vi "TCP.IP Server for Ripple Detection_requirements.vi"() -> ()   [LabVIEW 2021]
doc: "Demonstrates how to set up a basic TCP connection, send data to the specified port once a connection has been established, and terminate the connection once the data has been sent. This VI is designed to stop if the TCP connection is terminated. The data sent in this example is an array of random numbers."
panel:
  out "size":i64 format="%.6p"
  out "error IO":errorcluster
  in  "Number of row to read \nat a time":i32=10000
  in  "File Path":path
  out "Iteration terminal":i32
  in  "Stop 2":bool
  in  "Client Closed":string="The client VI closed the connection."
  in  "Stop":bool
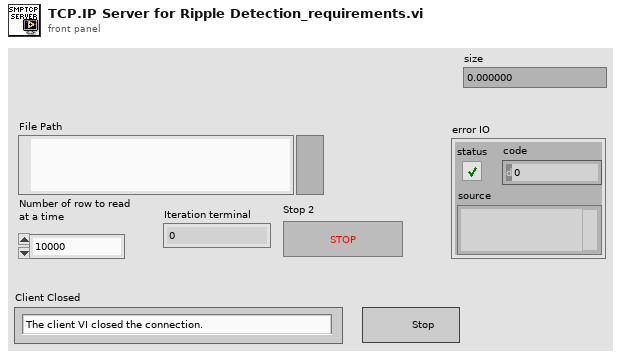
[diagram p1: front panel]
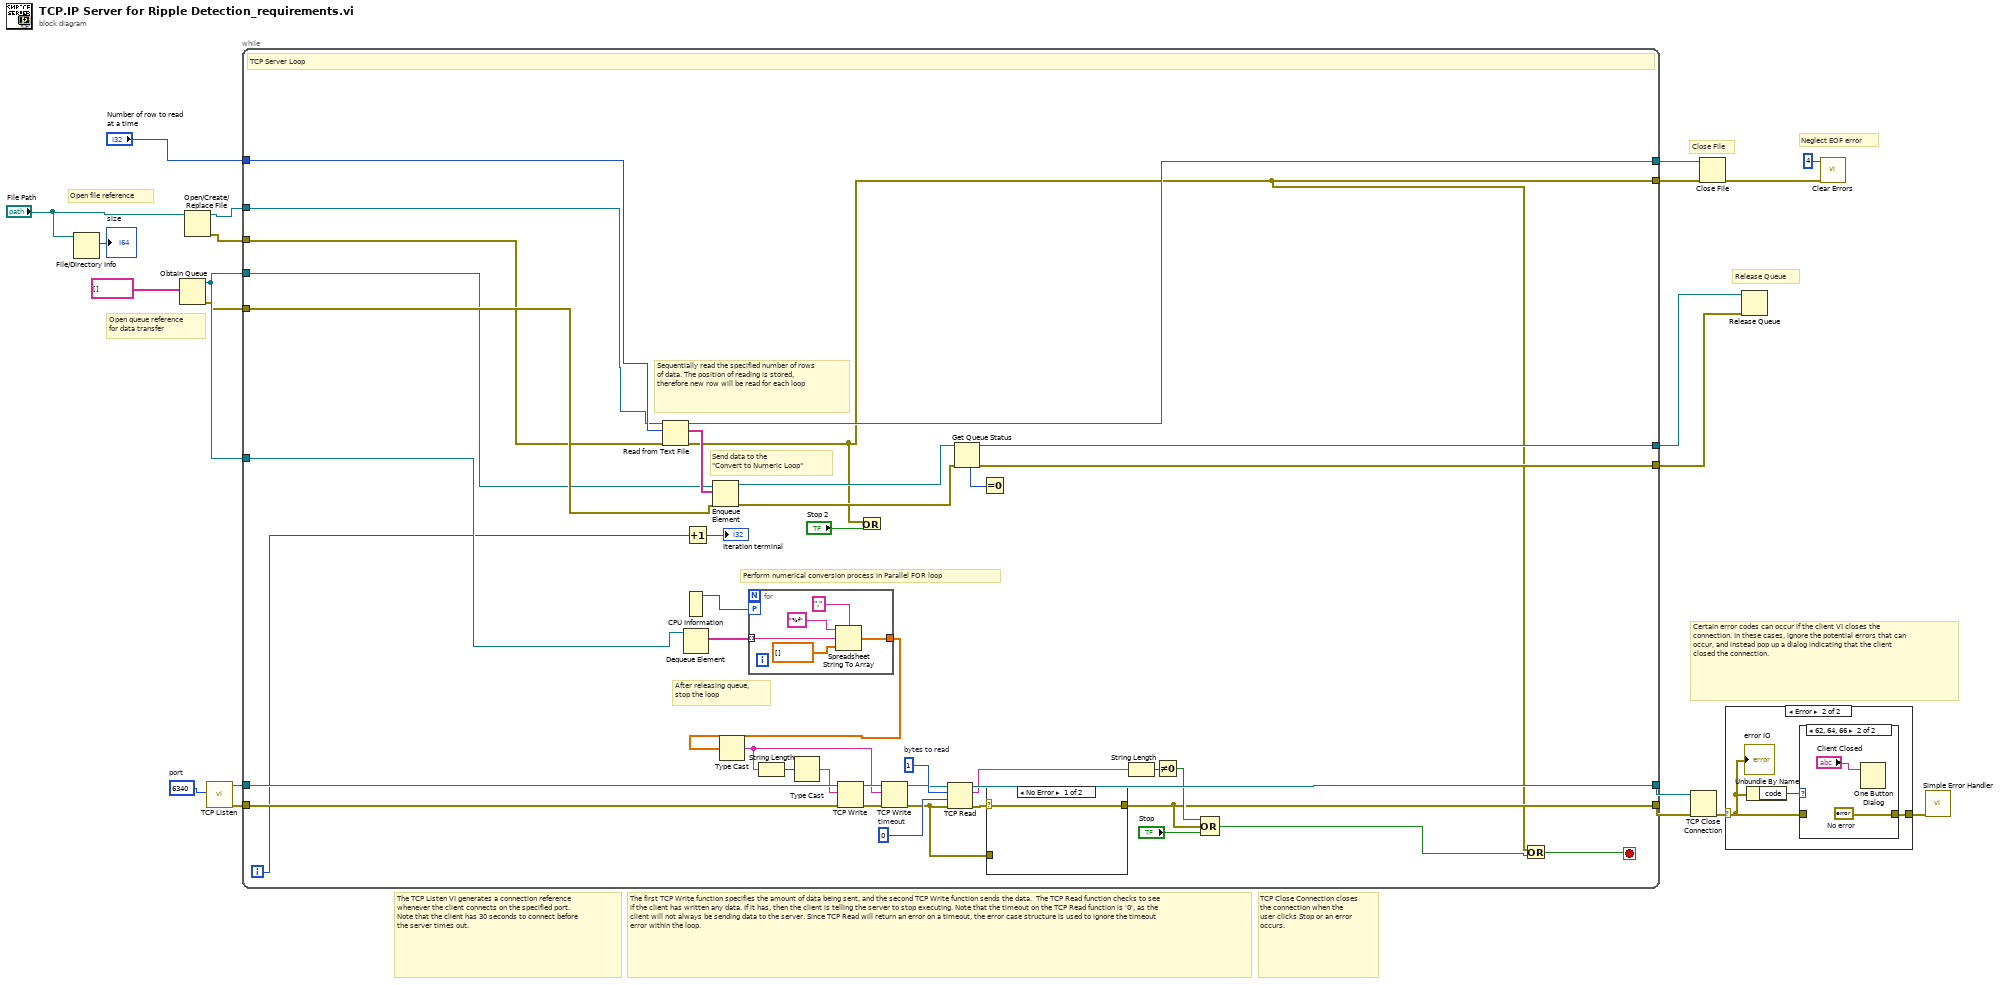
[diagram p0: block diagram]
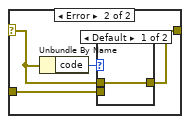
[diagram p4: hidden frame]
diagram:
  w15 = u16 6340  # port
  # "Neglect EOF error"
  # "Close File"
  # "Open queue reference\nfor data transfer"
  # "Release Queue"
  # "Open file reference"
  # "TCP Close Connection closes the connection when the user clicks Stop or an error occurs."
  # "The TCP Listen VI generates a connection reference whenever the client connects on the specified port. Note that the client has 30 seconds to connect before the server times out."
  # "Certain error codes can occur if the client VI closes the connection. In these cases, ignore the potential errors that can occur, and instead pop up a dialog indicating that the client closed the connection."
  # "The first TCP Write function specifies the amount of data being sent, and the second TCP Write function sends the data.  The TCP Read function checks to see if the client has written any data. If it has, then the client is telling the server to stop executing. Note that the timeout on the TCP Read function is '0', as the client will not always be sending data to the server. Since TCP Read will return an error on a timeout, the error case structure is used to ignore the timeout error within the loop."
  n1 = File/Directory Info(path="File Path") -> (size=→"size":i64)  [unwired: 1 in, 6 out]
  n2 = Obtain Queue(element data type=string[] [] ("形式文字列")) -> (queue out=w13:refnum<queue>, error out=w12:errorcluster)  [unwired: 4 in, 1 out]
  n3 = Open/Create/Replace File(file path (use dialog)="File Path") -> (refnum out=w1:refnum<file>, error out=w2:errorcluster)  [unwired: 5 in, 1 out]
  n4 = call <vilib>:"TCP Listen.vi"("port"=w15) -> ("error out"=w16:errorcluster, "connection ID"=w17:refnum<k5>)  [unwired: 6 in, 3 out]
  n5 = while {
    tunnel: [w45] -> w20
    tunnel: [w51] -> w21
    tunnel: w17 -> [w61]
    tunnel: w16 -> [w55]
    tunnel: w1 -> [w22]
    tunnel: w2 -> [w32]
    tunnel: w13 -> [w41]
    tunnel: w13 -> [w31]
    tunnel: w12 -> [w35]
    tunnel: "Number of row to read \nat a time" -> [w33]
    tunnel: [w29] -> w10
    tunnel: [w28] -> w9
    tunnel: [w24] -> w7
    tunnel: [w25] -> w6
    i -> [w34]
    stop <- w23 stop-if-true
    w50 = 0  # timeout
    w53 = 1  # bytes to read
    # "Send data to the \n\"Convert to Numeric Loop\""
    # "Sequentially read the specified number of rows of data. The position of reading is stored, therefore new row will be read for each loop"
    # "After releasing queue,\nstop the loop"
    # "Perform numerical conversion process in Parallel FOR loop"
    # "TCP Server Loop"
    n6 = Read from Text File(file (use dialog)=w22, count=w33, error in=w32) -> (refnum out=w25:refnum<file>, text=w38:string[], error out=w24:errorcluster)  [unwired: 1 in, 1 out]
    n7 = CPU Information() -> (4:w43:i32)  [unwired: 3 out]
    n8 = Dequeue Element(queue=w41) -> (element=w42:string[])  [unwired: 2 in, 3 out]
    n9 = Increment(x=w34) -> (x+1=→"Iteration terminal":i32)
    n10 = Enqueue Element(queue=w31, element=w38, error in (no error)=w35) -> (queue out=w30:refnum<queue>, error out=w27:errorcluster)  [unwired: 1 in, 1 out]
    n11 = for "Forループ" {
      tunnel: w42 -> [w63] mode=indexing
      tunnel: [w64] -> w40
      workers-P: w43 -> [_]
      n12 = Spreadsheet String To Array(delimiter (Tab)="," ("デリミタ（タブ）"), format string="%f" ("形式文字列"), spreadsheet string=w63, array type (2D Dbl)=dbl[] []) -> (array=w64:dbl[])
    }
    n13 = Type Cast(x=w40) -> (*(type *) &x=w56:string)  [unwired: 1 out]
    n14 = String Length(string=w56) -> (length=w58:i32)
    n15 = Type Cast(x=w58) -> (*(type *) &x=w57:string)  [unwired: 1 out]
    n16 = TCP Write(connection ID=w61, data in=w57, error in (no error)=w55) -> (connection ID out=w60:refnum<k5>, error out=w59:errorcluster)  [unwired: 2 out]
    n17 = Or(x=w24, y="Stop 2") -> ()  [unwired: 1 out]
    n18 = TCP Write(connection ID=w60, data in=w56, error in (no error)=w59) -> (connection ID out=w52:refnum<k5>, error out=w44:errorcluster)  [unwired: 2 out]
    n19 = TCP Read(connection ID=w52, bytes to read=w53, error in (no error)=w44, 9:w50) -> (connection ID out=w51:refnum<k5>, data out=w48:string, error out=w46:errorcluster)  [unwired: 1 out]
    n20 = Get Queue Status(queue=w30, error in (no error)=w27) -> (queue out=w29:refnum<queue>, error out=w28:errorcluster, # elements in queue=w36:i32)  [unwired: 1 in, 5 out]
    n21 = Equal To 0?(x=w36) -> ()  [unwired: 1 out]
    n22 = case shown="No Error" w46 {
      selector: w46 -> [w67 w70]
      tunnel: [w67 w68] -> w45
      tunnel: w44 -> [_ w69]
      frame No Error {
      }
      frame Error {
        n23 = Unbundle By Name(w70) -> ("code"=w71:i32)
        n24 = case shown="Default" w71 {
          tunnel: w70 -> [w72 _]
          tunnel: w69 -> [_ w73]
          tunnel: [w72 w73] -> w68
          frame Default {
          }
          frame 56 {
          }
        }
      }
    }
    n25 = String Length(string=w48) -> (length=w49:i32)
    n26 = Not Equal To 0?(x=w49) -> (x != 0?=w47:bool)
    n27 = Compound Arithmetic op=OR(w47, w45, "Stop") -> (w26:bool)
    n28 = Or(x=w24, y=w26) -> (x .or. y?=w23:bool)
  }
  n29 = TCP Close Connection(connection ID=w21, error in (no error)=w20) -> (error out=w19:errorcluster)  [unwired: 2 out]
  n30 = Close File(refnum=w6, error in=w7) -> (error out=w8:errorcluster)  [unwired: 1 out]
  n31 = case shown="Error" w19 {
    selector: w19 -> [w74 w76]
    tunnel: [w74 w75] -> w18
    frame No Error {
    }
    frame Error {
      n32 = Unbundle By Name(w76) -> ("code"=w77:i32)
      n33 = case shown="62, 64, 66" w77 {
        tunnel: w76 -> [w78 _]
        tunnel: [w78 w80] -> w75
        frame Default {
        }
        frame 62, 64, 66 {
          w80 = errorcluster {"status"=FALSE, "code"=0, "source"=""}  # No error
          n34 = One Button Dialog(message="Client Closed") -> ()  [unwired: 1 in, 1 out]
        }
      }
      "error IO" <- w76
    }
  }
  n35 = Release Queue(queue=w10, error in (no error)=w9) -> ()  [unwired: 1 in, 3 out]
  n36 = call <vilib>:"Clear Errors.vi"("error in (no error)"=w8, "specific error code to clear (0: all)"=4) -> ()  [unwired: 4 in, 2 out]
  n37 = call <vilib>:"Simple Error Handler.vi"("error in (no error)"=w18) -> ()  [unwired: 1 in, 8 out]
